vi "IsAtApartment.vi"() -> ()   [LabVIEW 2018]
panel:
  out "name":string
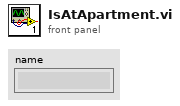
[diagram p1: front panel]
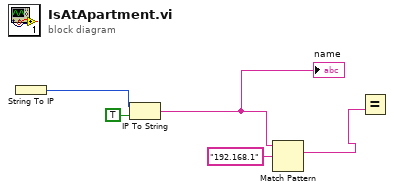
[diagram p0: block diagram]
diagram:
  n1 = String To IP() -> (0:w4:u32)  [unwired: 1 in]
  n2 = IP To String(1:TRUE ("dot notation? (F)"), 2:w4) -> (0:w3:string)
  "name" <- w3
  n3 = Match Pattern(string=w3, regular expression="192.168.1") -> (match substring=w1:string)  [unwired: 1 in, 3 out]
  n4 = Equal?(y=w1) -> ()  [unwired: 1 in, 1 out]
